vi "test11-RegisterUnregister_Event.vi"(8 "error in (no error)":errorcluster, 11 "TestCase in":refnum<class "testcase-CSMGlobalLog.lvclass">) -> (0 "error out":errorcluster, 3 "TestCase out":refnum<class "testcase-CSMGlobalLog.lvclass">)   [LabVIEW 2017, in "testcase-CSMGlobalLog.lvclass"]
uses:
  testcase-CSMGlobalLog.lvclass
  testcase-CSMGlobalLog.lvclass/testcase-CSMGlobalLog.ctl
  src/user.lib/_NEVSTOP/Communicable State Machine(CSM)/_Support/Typedef/_CSM_GlobalLog_MSG.ctl
  src/user.lib/_NEVSTOP/Communicable State Machine(CSM)/_Support/Typedef/_CSM_Response Source Message.ctl
  src/user.lib/_NEVSTOP/Communicable State Machine(CSM)/_Support/Typedef/_CSM_GlobalLog_MSG_TYPE.ctl
  936fda05-6a3c-48ea-a29d-4ce376580310.vi
  c0dc643a-0362-49fc-99f4-5251266ba5a0.vi
  src/user.lib/_NEVSTOP/Communicable State Machine(CSM)/_Support/GlobalEvent/GEvt-Generate with Rule Check.vi
  src/user.lib/_NEVSTOP/Communicable State Machine(CSM)/AdvanceAPI/CSM - Convert Error to Argument.vi
  src/user.lib/_NEVSTOP/Communicable State Machine(CSM)/_Support/GlobalEvent/Cache-GEvt Refs.vi
  src/user.lib/_NEVSTOP/Communicable State Machine(CSM)/AdvanceAPI/CSM - Make String Arguments Safe.vi
  src/user.lib/_NEVSTOP/Communicable State Machine(CSM)/_Support/ChangeFlag/FlagInstance-GEvt Refs.vi
  src/user.lib/_NEVSTOP/Communicable State Machine(CSM)/AdvanceAPI/CSM - Keywords.vi
  src/user.lib/_NEVSTOP/Communicable State Machine(CSM)/_Support/ChangeFlag/ChangeFlag-Read.vi
  src/user.lib/_NEVSTOP/Communicable State Machine(CSM)/_Support/ChangeFlag/ChangeFlagDB.vi
  src/user.lib/_NEVSTOP/Communicable State Machine(CSM)/_Support/GlobalEvent/FGV-GlobalEventRef(lvlibp).vi
  src/user.lib/_NEVSTOP/Communicable State Machine(CSM)/_Support/GlobalEvent/FGV-GlobalEventQueues(lvlibp).vi
  src/user.lib/_NEVSTOP/Communicable State Machine(CSM)/_Support/GlobalEvent/GEvt-Valid Subscribers.vi
  src/user.lib/_NEVSTOP/Communicable State Machine(CSM)/_Support/GlobalEvent/LogFilter/LogFilter - Check.vi
  src/user.lib/_NEVSTOP/Communicable State Machine(CSM)/_Support/GlobalEvent/LogFilter/LogFilter.lvclass
  <vilib>/addons/_JKI Toolkits/VI Tester/TestCase.llb/TestCase.lvclass
  src/user.lib/_NEVSTOP/Communicable State Machine(CSM)/Communicable State Machine.lvlib
  C:/Program Files (x86)/National Instruments/LabVIEW 2017/vi.lib/addons/_JKI Toolkits/VI Tester/TestCase.llb/TestCase.lvclass
panel:
  out "String cache each loop":string
  out "LoopCount":i32
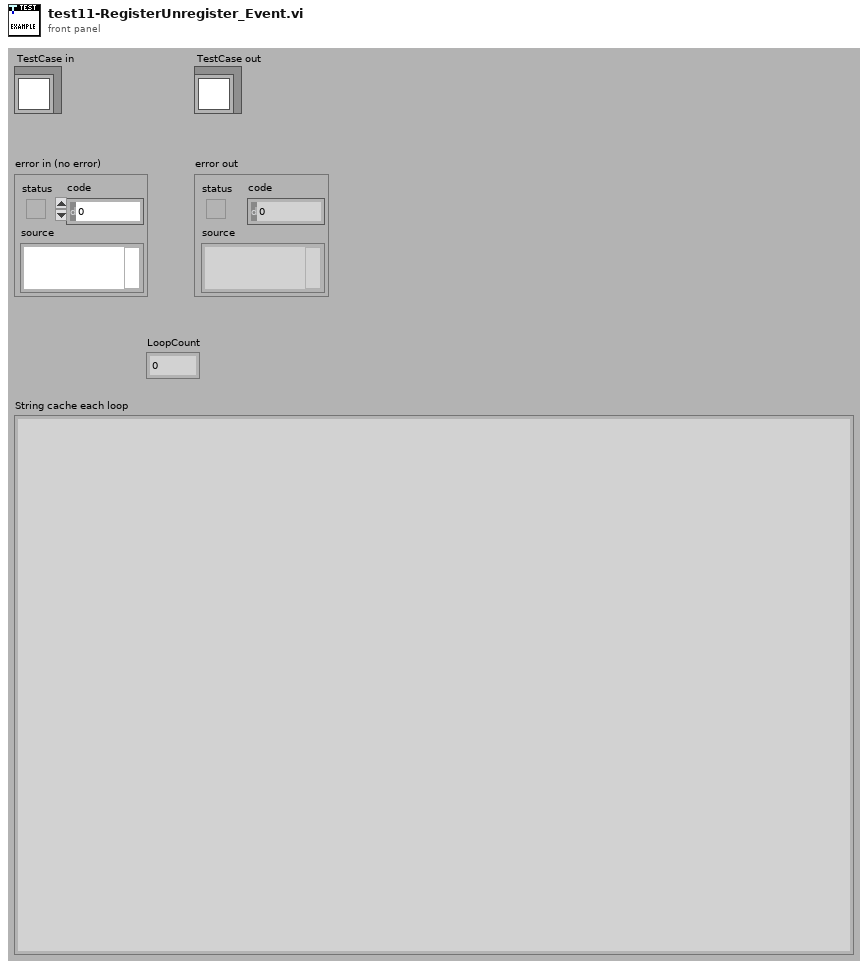
[diagram p1: front panel]
types:
  T1 = typedef "Communicable State Machine.lvlib/_CSM_GlobalLog_MSG.ctl" = cluster{"Name (\"\" to Use UUID)":string, "Current State":string, "Arguments":string, "Source Message":T2, "Source Module":string, "Complete(T)/Start(F)":bool, "LogType":T3, "Time Stamp":timestamp}
  T2 = typedef "Communicable State Machine.lvlib/_CSM_Response Source Message.ctl" = cluster{"‘State":string, "’Arguments":string, "’Error":errorcluster}
  T3 = typedef "Communicable State Machine.lvlib/_CSM_GlobalLog_MSG_TYPE.ctl" = enum16{"User Log", "State Change", "Status", "Interrupt", "Register", "Unregister", "Error Log", "Module Created", "Module Destroyed", "Async Message", "No-Rep Async Message", "Sync Message"}
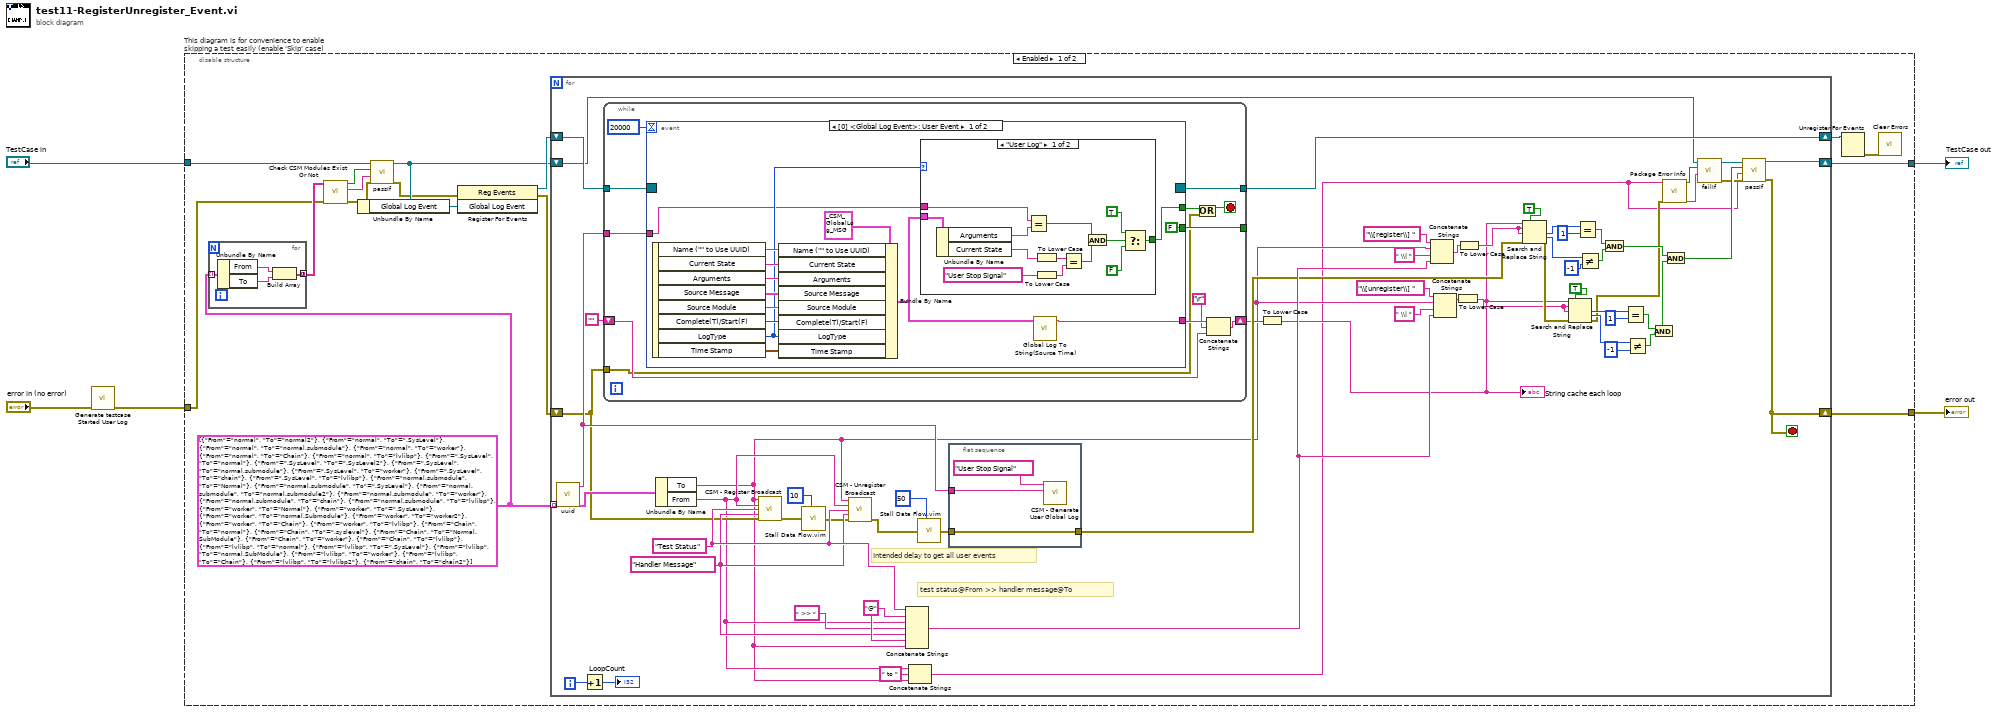
[diagram p0: block diagram]
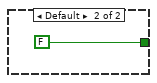
[diagram p2: hidden frame]
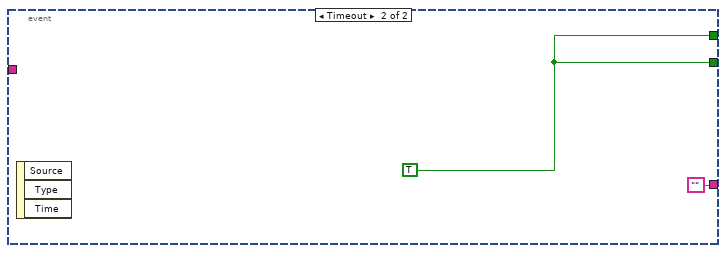
[diagram p3: hidden frame]
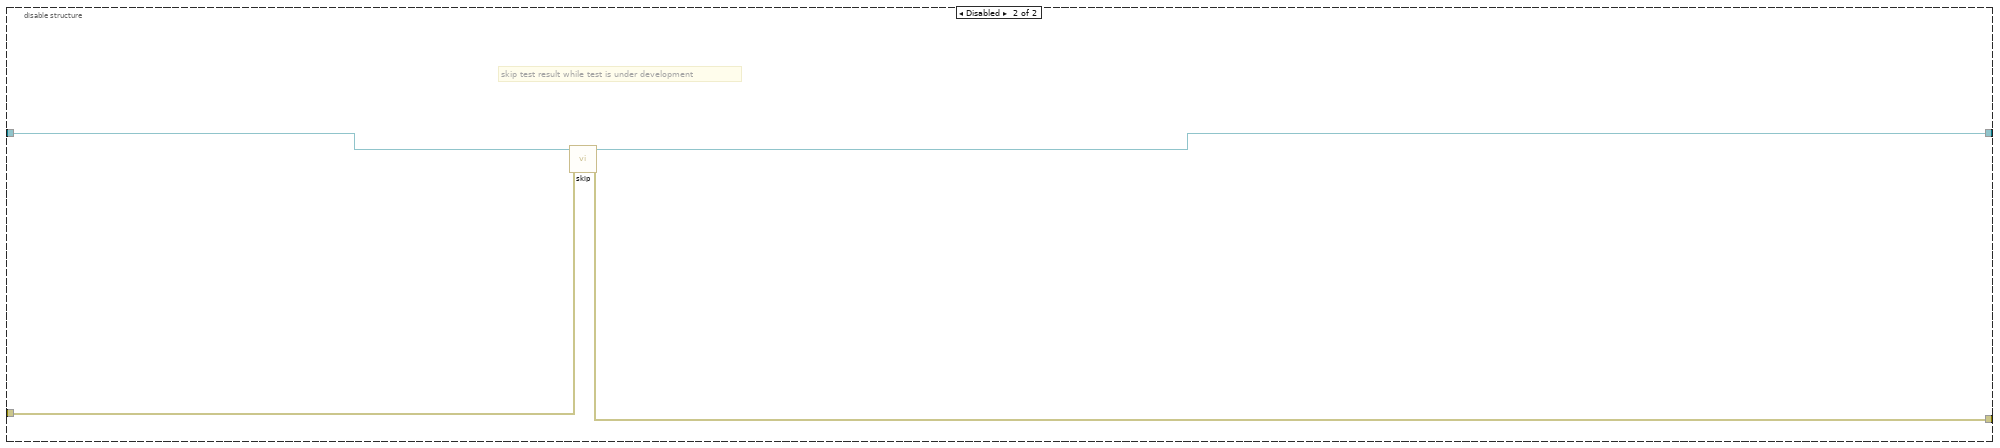
[diagram p4: hidden frame]
diagram:
  n1 = call "Generate testcase Started User Log.vi"("Error In"="error in (no error)") -> ("error out"=w1:errorcluster)  [unwired: 10 in]
  n2 = disable-structure "This diagram is for convenience to enable skipping a test easily (enable 'Skip' case)" shown="Enabled" {
    disable-tunnel: "TestCase in" -> [w9 w134]
    disable-tunnel: [w17 w132] -> w2
    disable-tunnel: [w16 w133] -> w4
    disable-tunnel: w1 -> [w10 w131]
    frame Enabled {
      w11 = cluster{"From":string, "To":string}[] [{"From"="normal", "To"="normal2"}, {"From"="normal", "To"=".SysLevel"}, {"From"="normal", "To"="normal.submodule"}, {"From"="normal", "To"="worker"}, {"From"="normal", "To"="Chain"}, {"From"="normal", "To"="lvlibp"}, {"From"=".SysLevel", "To"="normal"}, {"From"=".SysLevel", "To"=".SysLevel2"}, {"From"=".SysLevel", "To"="normal.submodule"}, {"From"=".SysLevel", "To"="worker"}, {"From"=".SysLevel", "To"="chain"}, {"From"=".SysLevel", "To"="lvlibp"}, {"From"="normal.submodule", "To"="Normal"}, {"From"="normal.submodule", "To"=".SysLevel"}, {"From"="normal.submodule", "To"="normal.submodule2"}, {"From"="normal.submodule", "To"="worker"}, {"From"="normal.submodule", "To"="chain"}, {"From"="normal.submodule", "To"="lvlibp"}, {"From"="worker", "To"="Normal"}, {"From"="worker", "To"=".SysLevel"}, {"From"="worker", "To"="normal.Submodule"}, {"From"="worker", "To"="worker2"}, {"From"="worker", "To"="Chain"}, {"From"="worker", "To"="lvlibp"}, {"From"="Chain", "To"="normal"}, {"From"="Chain", "To"=".syslevel"}, {"From"="Chain", "To"="Normal.SubModule"}, {"From"="Chain", "To"="worker"}, {"From"="Chain", "To"="lvlibp"}, {"From"="lvlibp", "To"="normal"}, {"From"="lvlibp", "To"=".SysLevel"}, {"From"="lvlibp", "To"="normal.SubModule"}, {"From"="lvlibp", "To"="worker"}, {"From"="lvlibp", "To"="Chain"}, {"From"="lvlibp", "To"="lvlibp2"}, {"From"="chain", "To"="chain2"}]
      n3 = for {
        tunnel: w11 -> [w25] mode=indexing
        tunnel: [w22] -> w14 mode=concatenating
        n4 = Unbundle By Name(w25) -> ("From"=w24:string, "To"=w23:string)
        n5 = Build Array(w24, w23) -> (w22:string[])
      }
      n6 = call "Check CSM Modules Exist Or Not.vi"("error in"=w10, "CSM names in"=w14) -> ("error out"=w12:errorcluster, "Debug string"=w13:string, "All Modules Exist?"=w15:bool)  [unwired: 7 in]
      n7 = call-dynamic "passIf.vi"("error in (no error)"=w12, "message (\"\")"=w13, "pass"=w15, "TestCase in"=w9) -> ("error out"=w7:errorcluster, "TestCase out"=w8:refnum<class "testcase-CSMGlobalLog.lvclass">)  [unwired: 6 in]
      n8 = Unbundle By Name(w8) -> ("Global Log Event"=w21:refnum<user-event>)
      n9 = register-events(error in=w7, w21) -> (reference out=w20:refnum<event-registration>, error out=w18:errorcluster)  [unwired: 1 in]
      n10 = for {
        shift-right: [w84] -> w19
        shift-left: w20 -> [w85]
        shift-right: [w81] -> w16
        shift-left: w18 -> [w40]
        tunnel: w11 -> [w49] mode=indexing
        shift-right: [w83] -> w17
        shift-left: w8 -> [w37]
        i -> [w44]
        stop <- w81 stop-if-true
        w61 = "@" ("Trigger")
        w59 = "Handler Message" ("API (If \"\", Same as Trigger)")
        w62 = "Test Status" ("Trigger")
        # "Intended delay to get all user events"
        # "test status@From >> handler message@To"
        n11 = call "uuid.vi"() -> ("UUID"=w46:string)  [unwired: 11 in]
        n12 = Increment(x=w44) -> (x+1=→"LoopCount":i32)
        n13 = while {
          tunnel: w85 -> [w100]
          tunnel: [w99] -> w84
          shift-right: [w92] -> w45
          shift-left: "" -> [w95]
          tunnel: w46 -> [w97]
          tunnel: [w96] -> _
          tunnel: w40 -> [w89]
          stop <- w91 stop-if-true
          n14 = event shown="[0] <Global Log Event>: User Event" {
            selector: w100 -> [_ _]
            dyn-events: [_ _] -> w99
            timeout: 20000 -> [_ _]
            tunnel: [w101 ""] -> w94
            tunnel: [w103 w130] -> w90
            tunnel: w97 -> [w104 _]
            tunnel: [FALSE ("Stop") w130] -> w96
            event User Event {
              n15 = event-data() -> ("Name (\"\" to Use UUID)"=w113:string, "Current State"=w112:string, "Arguments"=w111:string, "Source Message"=w110:T2, "Source Module"=w109:string, "Complete(T)/Start(F)"=w108:bool, "LogType"=w105:T3, "Time Stamp"=w107:timestamp)  [unwired: 1 in]
              n16 = Bundle By Name(cluster=T1 {"Name (\"\" to Use UUID)"="", "Current State"="", "Arguments"="", "Source Message"={"‘State"="", "’Arguments"="", "’Error"={"status"=FALSE, "code"=0, "source"=""}}, "Source Module"="", "Complete(T)/Start(F)"=FALSE, "LogType"=enum."State Change", "Time Stamp"=timestamp(0 s since 1904-01-01)} ("Cross CSM Data"), "Name (\"\" to Use UUID)"=w113, "Current State"=w112, "Arguments"=w111, "Source Message"=w110, "Source Module"=w109, "Complete(T)/Start(F)"=w108, "LogType"=w105, "Time Stamp"=w107) -> (w102:T1)
              n17 = case shown="\"User Log\"" w105 {
                tunnel: w102 -> [w127 _]
                tunnel: w104 -> [w126 _]
                tunnel: [w115 FALSE] -> w103
                frame "User Log" {
                  n18 = Unbundle By Name(w127) -> ("Arguments"=w125:string, "Current State"=w124:string)
                  n19 = Equal?(x=w126, y=w125) -> (x = y?=w119:bool)
                  n20 = To Lower Case(string=w124) -> (all lower case string=w123:string)
                  n21 = To Lower Case(string="User Stop Signal" ("Log")) -> (all lower case string=w121:string)
                  n22 = Equal?(x=w123, y=w121) -> (x = y?=w120:bool)
                  n23 = And(x=w119, y=w120) -> (x .and. y?=w118:bool)
                  n24 = Select(t=TRUE, s=w118, f=FALSE) -> (s? t:f=w115:bool)
                }
                frame Default {
                }
              }
              n25 = call "Global Log To String(Source Time).vi"("Log"=w102) -> ("Log String"=w101:string)  [unwired: 9 in]
            }
            event Timeout {
              w130 = TRUE ("Stop")
              n26 = event-data() -> ()  [unwired: 1 in, 3 out]
            }
          }
          n27 = Or(x=w90, y=w89) -> (x .or. y?=w91:bool)
          n28 = Concatenate Strings(w94, "\r", w95) -> (w92:string)
        }
        n29 = Unbundle By Name(w49) -> ("To"=w32:string, "From"=w33:string)
        n30 = call "CSM - Register Broadcast.vi"("CSM Name(Empty for Broadcast Event)"=w32, "Source CSM Name (* as Default)"=w33, "Trigger"=w62, "API (If \"\", Same as Trigger)"=w59, "Error In"=w40) -> ("error out"=w28:errorcluster)  [unwired: 9 in, 1 out]
        n31 = call "Stall Data Flow.vim"("value in"=w28, "milliseconds to wait"=u32 10) -> ("value out"=w27:errorcluster)  [unwired: 1 out]
        n32 = call "CSM - Unregister Broadcast.vi"("CSM Name(Empty for Broadcast Event)"=w32, "Source CSM Name (* as Default)"=w33, "Trigger"=w62, "API (\"*\" as Default)"=w59, "Error In"=w27) -> ("error out"=w80:errorcluster)  [unwired: 9 in, 1 out]
        n33 = Concatenate Strings(w62, w61, w33, " >> " ("string"), w59, w61, w32) -> (w79:string)
        n34 = Concatenate Strings(w33, " to " ("string"), w32) -> (w30:string)
        n35 = call "Stall Data Flow.vim"("value in"=w80, "milliseconds to wait"=u32 50) -> ("value out"=w48:errorcluster)  [unwired: 1 out]
        n36 = flat-sequence {
          tunnel: w46 -> [w87]
          tunnel: w48 -> [w86]
          tunnel: [w86] -> w47
          frame #0 {
            n37 = call "CSM - Generate User Global Log.vi"("Arguments"=w87, "Log"="User Stop Signal") -> ()  [unwired: 9 in, 1 out]
          }
        }
        n38 = To Lower Case(string=w45) -> (all lower case string=w41:string)
        "String cache each loop" <- w41
        n39 = Concatenate Strings("\\[register\\] " ("regular expression"), w32, " \\| " ("string"), w79) -> (w65:string)
        n40 = Concatenate Strings("\\[unregister\\] " ("regular expression"), w32, " \\| " ("string"), w79) -> (w64:string)
        n41 = To Lower Case(string=w64) -> (all lower case string=w75:string)
        n42 = To Lower Case(string=w65) -> (all lower case string=w66:string)
        n43 = Search and Replace String(replace all?=TRUE ("replace all? (F)"), input string=w41, search string=w66, replace string=w66, error in=w47) -> (number of replacements=w67:i32, offset past replacement=w68:i32, error out=w76:errorcluster)  [unwired: 3 in, 1 out]
        n44 = Search and Replace String(replace all?=TRUE ("replace all? (F)"), input string=w41, search string=w75, replace string=w75, error in=w76) -> (number of replacements=w74:i32, offset past replacement=w73:i32, error out=w34:errorcluster)  [unwired: 3 in, 1 out]
        n45 = Equal?(x=w67, y=1) -> (x = y?=w69:bool)
        n46 = Not Equal?(x=w68, y=-1) -> (x != y?=w70:bool)
        n47 = And(x=w69, y=w70) -> (x .and. y?=w78:bool)
        n48 = Equal?(x=w74, y=1) -> (x = y?=w72:bool)
        n49 = Not Equal?(x=w73, y=-1) -> (x != y?=w71:bool)
        n50 = And(x=w72, y=w71) -> (x .and. y?=w77:bool)
        n51 = call "Package Error Info.vi"("error in"=w34, "String in"=w30) -> ("packed error info out"=w38:string, "error status"=w39:bool)  [unwired: 8 in]
        n52 = And(x=w78, y=w77) -> (x .and. y?=w43:bool)
        n53 = call-dynamic "failIf.vi"("message (\"\")"=w38, "fail"=w39, "TestCase in"=w37) -> ("error out"=w35:errorcluster, "TestCase out"=w36:refnum<class "testcase-CSMGlobalLog.lvclass">)  [unwired: 7 in]
        n54 = call-dynamic "passIf.vi"("error in (no error)"=w35, "message (\"\")"=w30, "pass"=w43, "TestCase in"=w36) -> ("error out"=w81:errorcluster, "TestCase out"=w83:refnum<class "testcase-CSMGlobalLog.lvclass">)  [unwired: 6 in]
      }
      n55 = Unregister For Events(event registration refnum=w19) -> (error out=w6:errorcluster)  [unwired: 1 in]
      n56 = call <vilib>:"Clear Errors.vi"("error in (no error)"=w6) -> ()  [unwired: 5 in, 2 out]
    }
    frame Disabled {
      # "skip test result while test is under development"
      n57 = call <vilib>:"skip.vi"("error in (no error)"=w131, "TestCase in"=w134) -> ("error out"=w133:errorcluster, "TestCase out"=w132:refnum<class "testcase-CSMGlobalLog.lvclass">)  [unwired: 8 in]
    }
  }
  "error out" <- w4
  "TestCase out" <- w2
